vi "ULx Create Channel (CI-Two Edge Separation).vi"(0 "task in":refnum<k24>, 5 "counters":refnum<k21>, 9 "units":i32(ring) items=["Seconds", "Ticks"], 11 "error in":errorcluster, 13 "first edge":i32(ring) items=["Rising", "Falling"], 14 "second edge":i32(ring) items=["Rising", "Falling"]) -> (4 "task out":refnum<k24>, 15 "error out":errorcluster)   [LabVIEW 2020]
doc: "Creates channel(s) to measure the period of digital signals."
uses:
  C:/Users/William/Documents/LV 2020 builds/LeaktestDAQ/Source-v33/ULx_LV.dll
  ULx_LV.dll
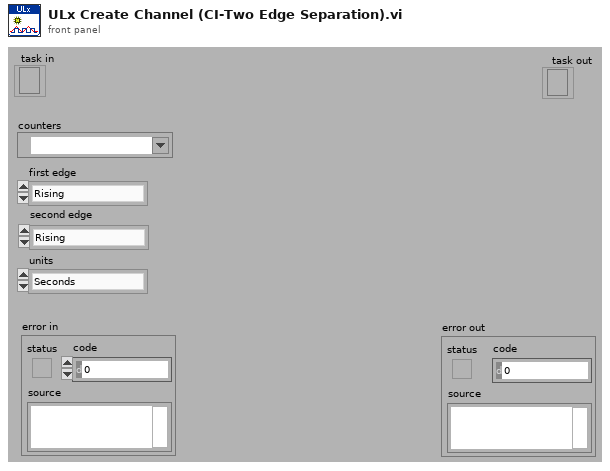
[diagram p1: front panel]
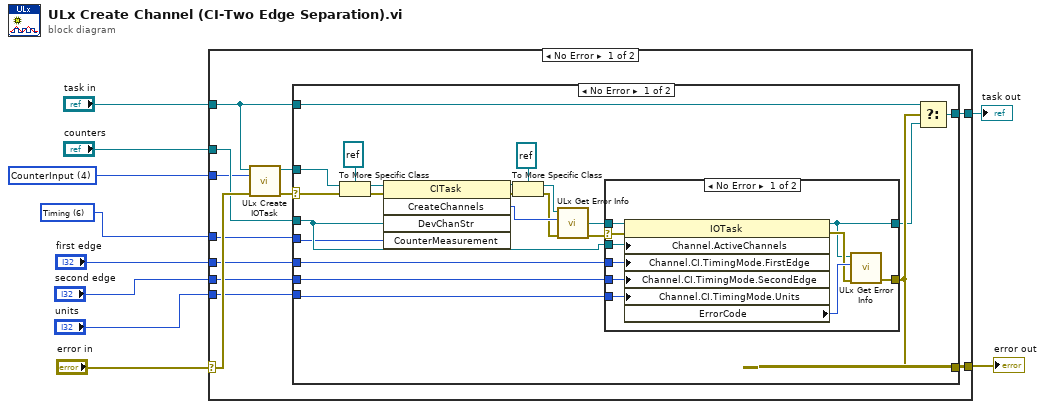
[diagram p0: block diagram]
diagram:
  w2 = 6 items=["CountEdges"=1, "Encoder"=2, "Frequency"=3, "Period"=4, "PulseWidth"=5, "Timing"=6] ("CounterMeasurement")
  w6 = 4 items=["AnalogInput", "AnalogOutput", "DigitalInput", "DigitalOutput", "CounterInput", "CounterOutput", "CompositeInput", "CompositeOutput", "TemperatureInput"] ("taskType")
  n1 = case shown="No Error" "error in" {
    selector: "error in" -> [w22 w59]
    tunnel: "task in" -> [w13 w58]
    tunnel: "counters" -> [w17 _]
    tunnel: [w20 w58] -> w8
    tunnel: [w19 w59] -> w7
    tunnel: w6 -> [w16 _]
    tunnel: "first edge" -> [w15 _]
    tunnel: "units" -> [w14 _]
    tunnel: w2 -> [w12 _]
    tunnel: "second edge" -> [w11 _]
    frame No Error {
      n2 = call "ULx Create IOTask.vi"("error in"=w22, "taskType"=w16, "i/o task in"=w13) -> ("error out"=w21:errorcluster, "i/o task out"=w18:refnum<k24>)  [unwired: 7 in]
      n3 = case shown="No Error" w21 {
        selector: w21 -> [w41 w57]
        tunnel: [w27 w57] -> w19
        tunnel: [w28 w56] -> w20
        tunnel: w18 -> [w39 _]
        tunnel: w17 -> [w36 _]
        tunnel: w15 -> [w35 _]
        tunnel: w14 -> [w34 _]
        tunnel: w13 -> [w25 w56]
        tunnel: w12 -> [w24 _]
        tunnel: w11 -> [w23 _]
        frame No Error {
          n4 = To More Specific Class(target class=refnum<k24> refnum, reference=w39, error in=w41) -> (specific class reference=w42:refnum<k24>, error out=w40:errorcluster)
          n5 = invoke class="CITask" method="CreateChannels"(reference=w42, error in=w40, "DevChanStr"=w36, "CounterMeasurement"=w24) -> (reference out=w32:refnum<k24>, error out=w31:errorcluster, "CreateChannels"=w38:i32)  [unwired: 1 in, 2 out]
          n6 = To More Specific Class(target class=refnum<k24> refnum, reference=w32, error in=w31) -> (specific class reference=w29:refnum<k24>, error out=w30:errorcluster)
          n7 = call "ULx Get Error Info.vi"("error in"=w30, "ErrorCode"=w38, "task in"=w29) -> ("error out"=w37:errorcluster)  [unwired: 8 in]
          n8 = case shown="No Error" w37 {
            selector: w37 -> [w53 w55]
            tunnel: w29 -> [w52 w54]
            tunnel: w36 -> [w51 _]
            tunnel: [w48 w55] -> w27
            tunnel: w35 -> [w47 _]
            tunnel: w34 -> [w46 _]
            tunnel: [w45 w54] -> w26
            tunnel: w23 -> [w44 _]
            frame No Error {
              n9 = property class="IOTask"(reference=w52, error in=w53, "Channel.ActiveChannels"=w51, "Channel.CI.TimingMode.FirstEdge"=w47, "Channel.CI.TimingMode.SecondEdge"=w44, "Channel.CI.TimingMode.Units"=w46) -> (reference out=w45:refnum<k24>, error out=w49:errorcluster, "ErrorCode"=w50:i32)
              n10 = call "ULx Get Error Info.vi"("error in"=w49, "ErrorCode"=w50, "task in"=w45) -> ("error out"=w48:errorcluster)  [unwired: 8 in]
            }
            frame Error {
            }
          }
          n11 = Select(t=w25, s=w27, f=w26) -> (s? t:f=w28:refnum<k24>)
        }
        frame Error {
        }
      }
    }
    frame Error {
    }
  }
  "error out" <- w7
  "task out" <- w8
